vi "Demo.vi"() -> ()   [LabVIEW 2018, in "LogonUser.lvclass"]
doc: "©2019\nWiebe Walstra\nwww.carya.nl"
uses:
  LogonUser.lvclass
  Threads.ctl
  a5da16ea-324e-4874-85ed-5cb7efe69a92.vi
  33f4221f-8772-43d3-a4c0-4406f15abd77.vi
  98d08e1c-2519-46bd-bc2e-7f1d875dff32.vi
  11e4732c-09a4-4816-9c4f-a717da3eb60a.vi
  kernel32.dll
panel:
  out "-1":i32
  out "1":i32
  out "should succeed":errorcluster
  out "should fail":errorcluster
  out "should succeed":errorcluster
  out "should succeed":errorcluster
  out "should fail":errorcluster
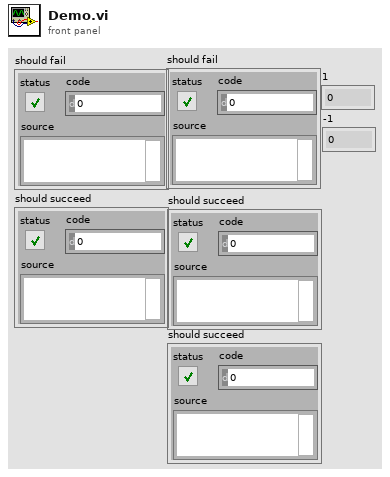
[diagram p1: front panel]
types:
  T1 = typedef "LogonUser.lvclass/Threads.ctl" = enum32{"user interface", "standard", "instrument i/o", "data acquisition", "other 1", "other 2", "same as caller", "manual"}
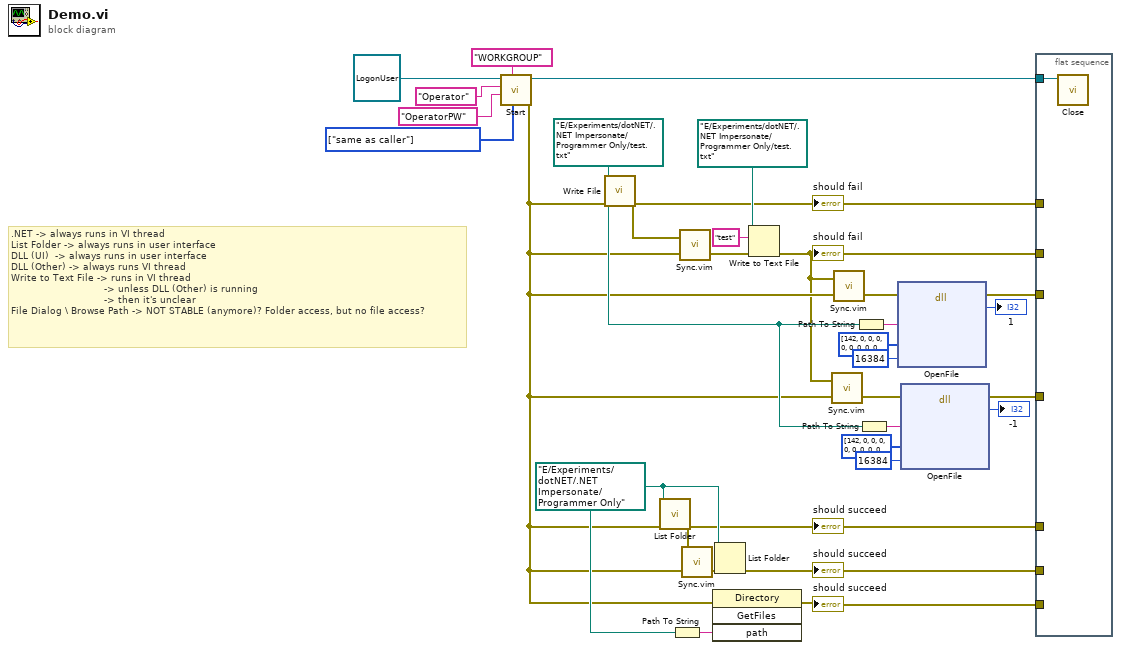
[diagram p0: block diagram]
diagram:
  w23 = path "E:/Experiments/dotNET/.NET Impersonate/Programmer Only" ("path")
  w17 = T1[] [enum."same as caller"] items=["user interface", "standard", "instrument i/o", "data acquisition", "other 1", "other 2", "same as caller", "manual"] ("Thread")
  w19 = path "E:/Experiments/dotNET/.NET Impersonate/Programmer Only/test.txt" ("path")
  # ".NET -> always runs in VI thread\nList Folder -> always runs in user interface\nDLL (UI)  -> always runs in user interface\nDLL (Other) -> always runs VI thread\nWrite to Text File -> runs in VI thread\n                               -> unless DLL (Other) is running\n                               -> then it's unclear\nFile Dialog \\ Browse Path -> NOT STABLE (anymore)? Folder access, but no file access?"
  n1 = call-dynamic "Start.vi"("Thread"=w17, "domainName"="WORKGROUP", "password"="OperatorPW", "userName"="Operator", "Impersonate in"=refnum<class "LogonUser.lvclass"> refnum) -> ("error out"=w4:errorcluster, "Impersonate out"=w30:refnum<class "LogonUser.lvclass">)  [unwired: 5 in]
  n2 = call "Write File.vi"("error in (no error)"=w4, "path"=w19) -> ("error out"=w1:errorcluster)  [unwired: 9 in]
  "should fail" <- w1
  n3 = call "List Folder.vi"("error in (no error)"=w4, "path"=w23) -> ("error out"=w6:errorcluster)  [unwired: 9 in]
  "should succeed" <- w6
  n4 = Path To String(path=w23) -> (string=w24:string)
  n5 = call "Sync.vim"("a"=w1, "b"=w4) -> ("b'"=w3:errorcluster)  [unwired: 24 in, 1 out]
  n6 = call "Sync.vim"("a"=w6, "b"=w4) -> ("b'"=w5:errorcluster)  [unwired: 24 in, 1 out]
  n7 = invoke class="Directory" method="GetFiles"(error in=w4, "path"=w24) -> (error out=w22:errorcluster)  [unwired: 2 in, 3 out]
  "should succeed" <- w22
  n8 = List Folder(path=w23, error in=w5) -> (error out=w26:errorcluster)  [unwired: 2 in, 3 out]
  "should succeed" <- w26
  n9 = Write to Text File(file (use dialog)=path "E:/Experiments/dotNET/.NET Impersonate/Programmer Only/test.txt" ("path"), text="test", error in=w3) -> (error out=w2:errorcluster)  [unwired: 1 in, 2 out]
  "should fail" <- w2
  n10 = call "Sync.vim"("a"=w2, "b"=w4) -> ("b'"=w8:errorcluster)  [unwired: 24 in, 1 out]
  n11 = call "Sync.vim"("a"=w2, "b"=w4) -> ()  [unwired: 24 in, 2 out]
  n12 = Path To String(path=w19) -> (string=w14:string)
  n13 = Path To String(path=w19) -> (string=w13:string)
  n14 = dll-call lib="kernel32.dll" fn="OpenFile"(error in=w4, "file"=w14, "lpReOpenBuff"=i32[] [142, 0, 0, 0, 0, 0, 0, 0, 0, 0, 0, 0, 0, 0, 0, 0, 0, 0, 0, 0, 0, 0, 0, 0, 0, 0, 0, 0, 0, 0, 0, 0, 0, 0, 0, 0, 0, 0, 0, 0, 0, 0, 0, 0, 0, 0, 0, 0, 0, 0, 0, 0, 0, 0, 0, 0, 0, 0, 0, 0, 0, 0, 0, 0, 0, 0, 0, 0, 0, 0, 0, 0, 0, 0, 0, 0, 0, 0, 0, 0, 0, 0, 0, 0, 0, 0, 0, 0, 0, 0, 0, 0, 0, 0, 0, 0, 0, 0, 0, 0, 0, 0, 0, 0, 0, 0, 0, 0, 0, 0, 0, 0, 0, 0, 0, 0, 0, 0, 0, 0, 0, 0, 0, 0, 0, 0, 0, 0, 0, 0, 0, 0, 0, 0, 0, 0, 0, 0, 0, 0, 0, 0], "uStyle"=16384) -> (error out=w20:errorcluster, "return type"=→"1":i32)  [unwired: 5 in, 1 out]
  n15 = dll-call lib="kernel32.dll" fn="OpenFile"(error in=w8, "file"=w13, "lpReOpenBuff"=i32[] [142, 0, 0, 0, 0, 0, 0, 0, 0, 0, 0, 0, 0, 0, 0, 0, 0, 0, 0, 0, 0, 0, 0, 0, 0, 0, 0, 0, 0, 0, 0, 0, 0, 0, 0, 0, 0, 0, 0, 0, 0, 0, 0, 0, 0, 0, 0, 0, 0, 0, 0, 0, 0, 0, 0, 0, 0, 0, 0, 0, 0, 0, 0, 0, 0, 0, 0, 0, 0, 0, 0, 0, 0, 0, 0, 0, 0, 0, 0, 0, 0, 0, 0, 0, 0, 0, 0, 0, 0, 0, 0, 0, 0, 0, 0, 0, 0, 0, 0, 0, 0, 0, 0, 0, 0, 0, 0, 0, 0, 0, 0, 0, 0, 0, 0, 0, 0, 0, 0, 0, 0, 0, 0, 0, 0, 0, 0, 0, 0, 0, 0, 0, 0, 0, 0, 0, 0, 0, 0, 0, 0, 0], "uStyle"=16384) -> (error out=w18:errorcluster, "return type"=→"-1":i32)  [unwired: 5 in, 1 out]
  n16 = flat-sequence {
    tunnel: w30 -> [w31]
    tunnel: w1 -> [_]
    tunnel: w2 -> [_]
    tunnel: w6 -> [_]
    tunnel: w26 -> [_]
    tunnel: w22 -> [_]
    tunnel: w20 -> [_]
    tunnel: w18 -> [_]
    frame #0 {
      n17 = call-dynamic "Close.vi"("Impersonate in"=w31) -> ()  [unwired: 9 in, 2 out]
    }
  }
